vi "Axsun OCT Control Example - revise.vi"() -> ()   [LabVIEW 2018]
uses:
  C:/Users/BoasLab/Downloads/AxsunOCTControlExampleSourceCode_LabVIEW/AxsunOCTControl.dll
  AxsunOCTControl.dll
panel:
  out "BytesSent":i32
  out "TimeTaken":i32
  out "PacketsSent":i32
  out "DataBytes":i32
  out "StatusArray":u32[](array[numeric])
  out "StatusWordsReturned":u32
  out "SerialNum":string
  out "SourceCurrentOn 2":u32
  out "LaserOnTimeSeconds":u32
  in  "GetSerialNum":bool
  in  "CloseConnection":bool
  in  "GetLastCommandInfo":bool
  in  "RebootSystem":bool
  in  "GetSystemStatus":bool
  in  "SourceCurrentOFF":bool
  in  "Initialize":bool
  in  "SourceCurrentOn":bool
  out "wavelength":dbl
  in  "GetWaveLengthAtSweepTrigger":bool
  in  "GetLaserOnTime":bool
  out "Devices":string[](array[string])
  in  "Laser Off":bool
  in  "Laser On":bool
  in  "stop":bool
  out "Error":errorcluster
  out "Version":string
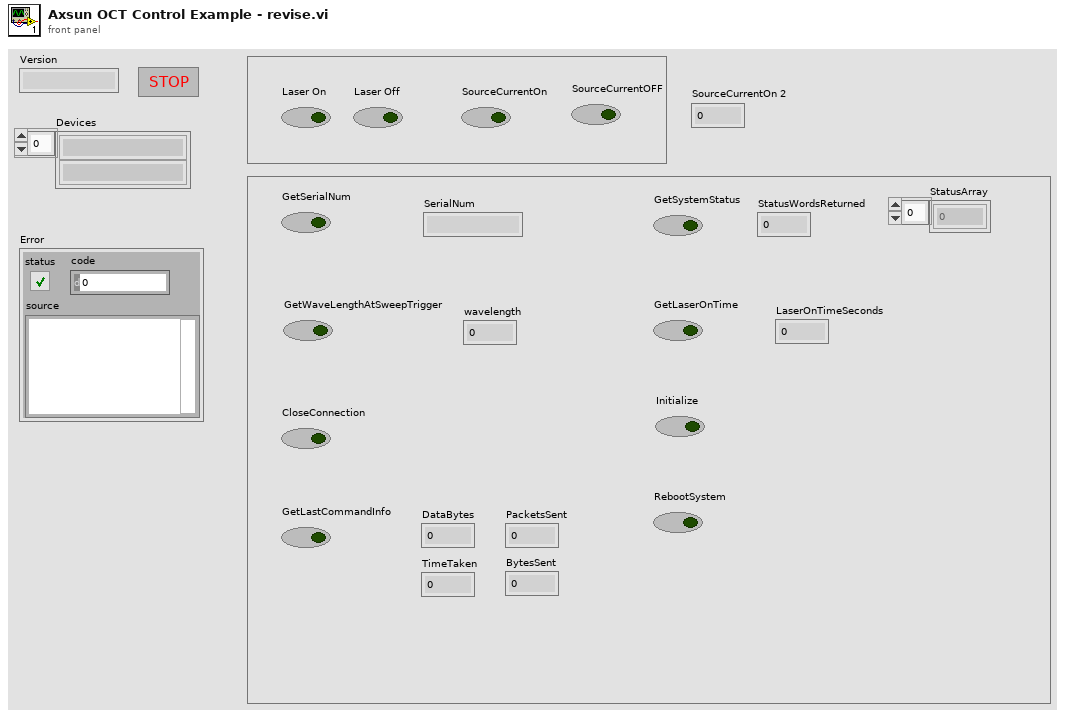
[diagram p1: front panel]
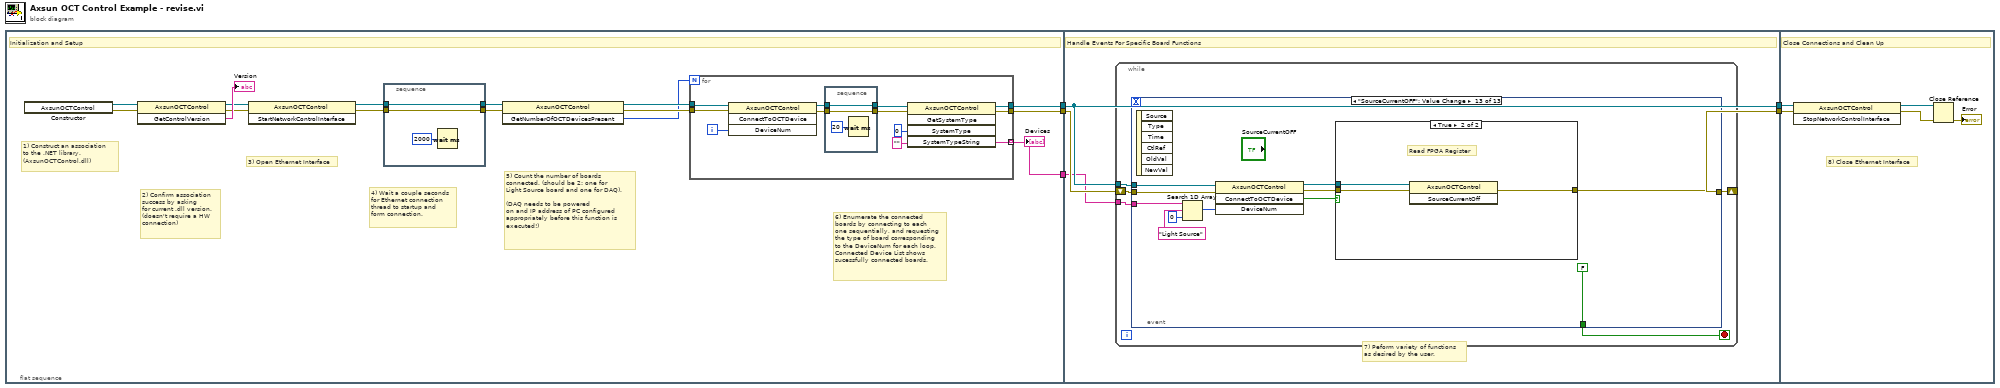
[diagram p0: block diagram]
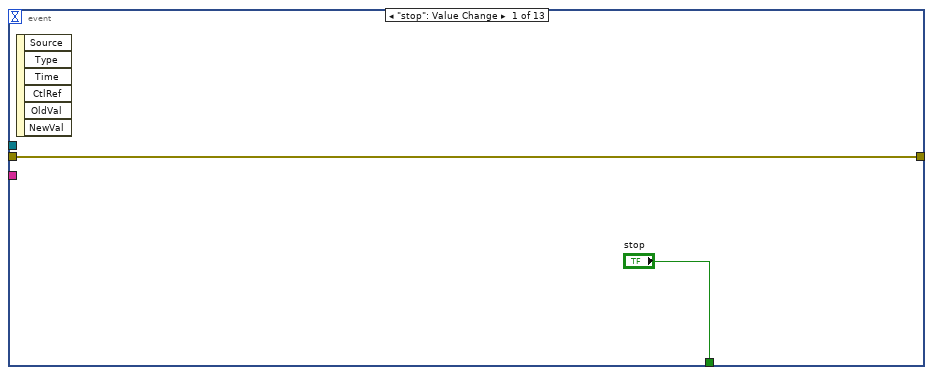
[diagram p2: hidden frame]
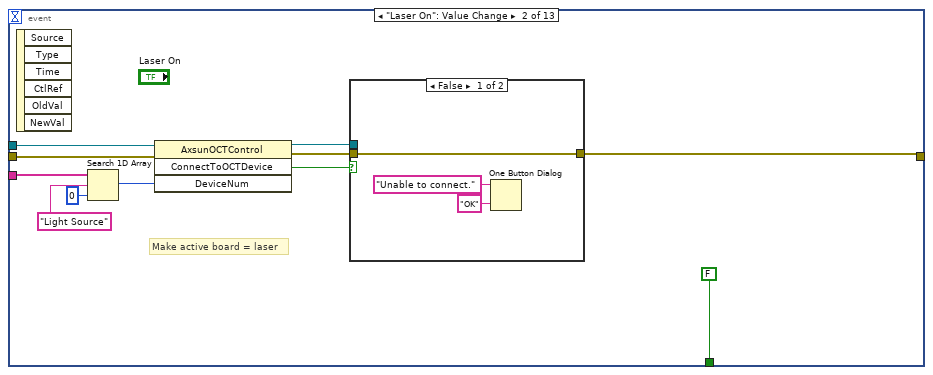
[diagram p3: hidden frame]
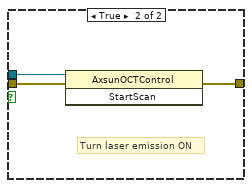
[diagram p4: hidden frame]
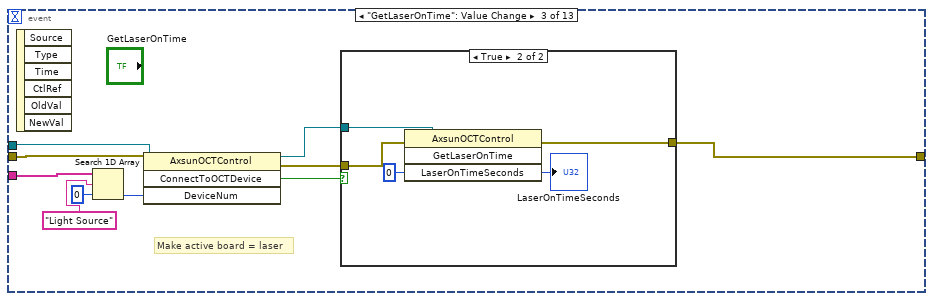
[diagram p5: hidden frame]
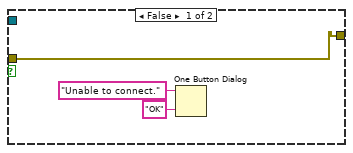
[diagram p6: hidden frame]
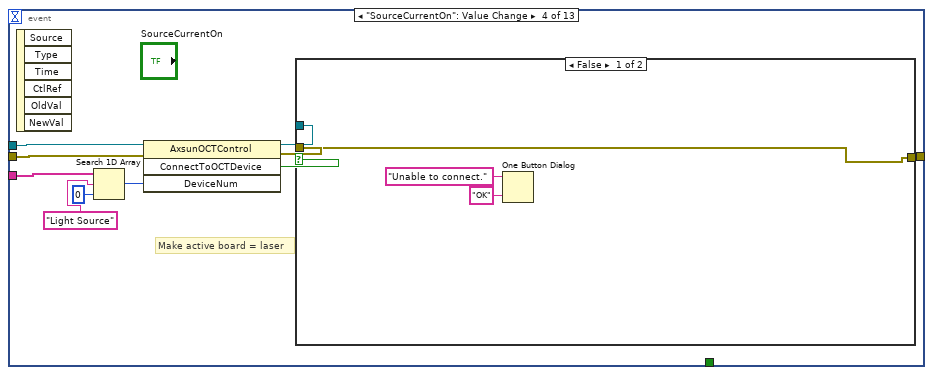
[diagram p7: hidden frame]
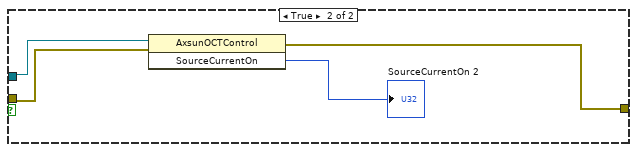
[diagram p8: hidden frame]
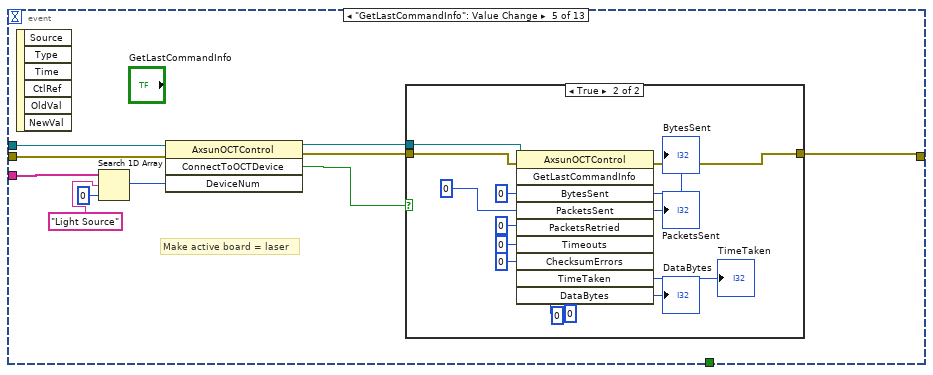
[diagram p9: hidden frame]
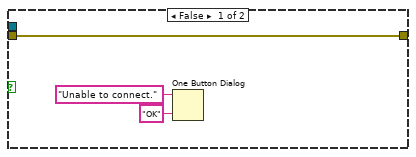
[diagram p10: hidden frame]
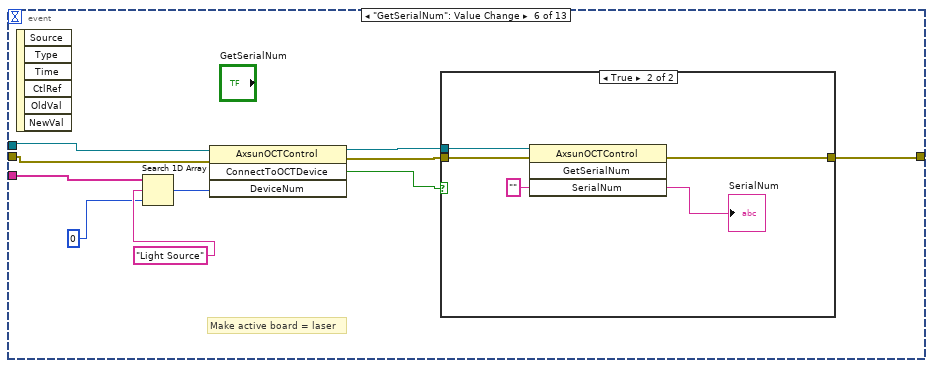
[diagram p11: hidden frame]
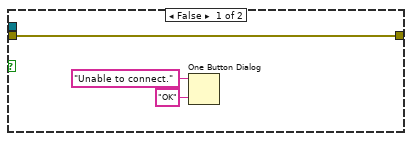
[diagram p12: hidden frame]
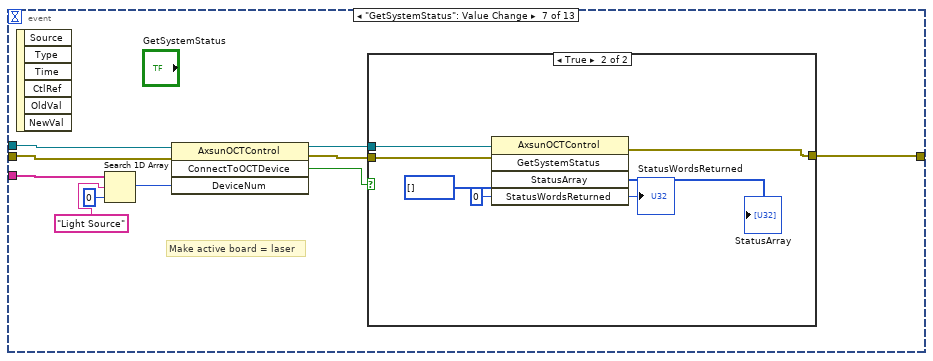
[diagram p13: hidden frame]
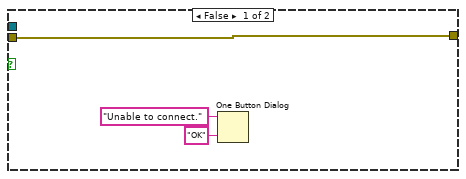
[diagram p14: hidden frame]
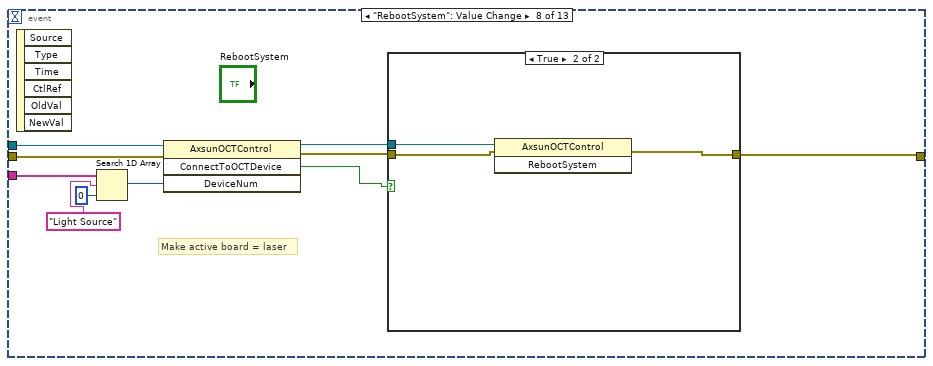
[diagram p15: hidden frame]
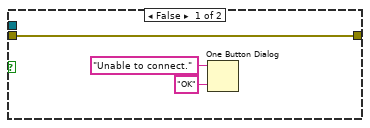
[diagram p16: hidden frame]
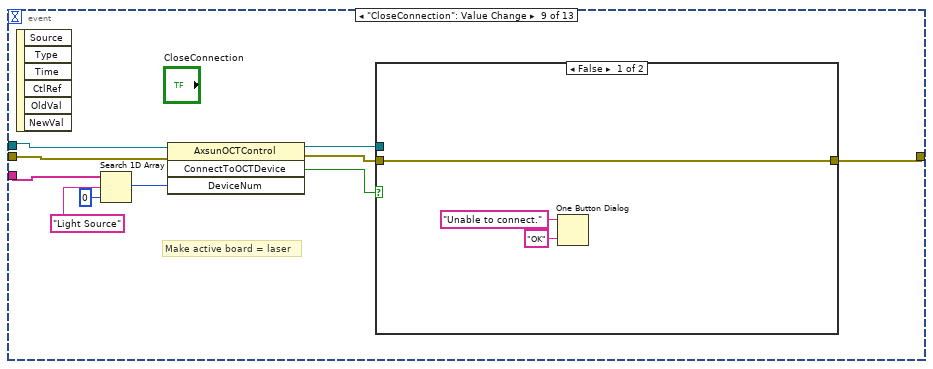
[diagram p17: hidden frame]
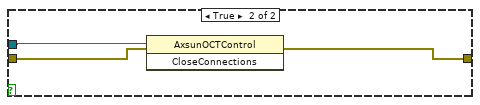
[diagram p18: hidden frame]
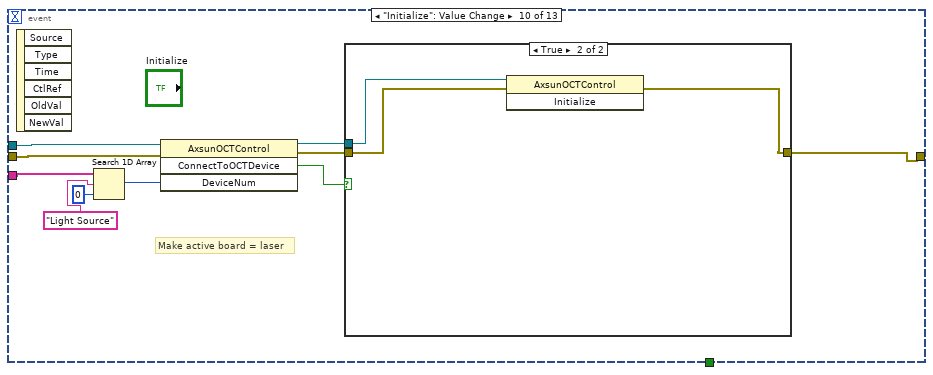
[diagram p19: hidden frame]
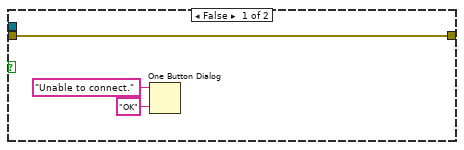
[diagram p20: hidden frame]
diagram:
  n1 = flat-sequence {
    tunnel: [w11] -> w5
    tunnel: [w10] -> w4
    tunnel: [w9] -> w2
    tunnel: w5 -> [w42]
    tunnel: w4 -> [w41]
    tunnel: [w41] -> w3
    tunnel: w2 -> [w40]
    tunnel: [w39] -> w1
    tunnel: w3 -> [w270]
    tunnel: w1 -> [w266]
    frame #0 {
      # "6) Enumerate the connected\nboards by connecting to each\none sequentially, and requesting\nthe type of board corresponding\nto the DeviceNum for each loop.\nConnected Device List shows\nsucessfully connected boards."
      # "5) Count the number of boards\nconnected. (should be 2: one for\nLight Source board and one for DAQ).\n\n(DAQ needs to be powered\non and IP address of PC configured \nappropriately before this function is\nexecuted!)"
      # "4) Wait a couple seconds\nfor Ethernet connection\nthread to startup and\nform connection."
      # "3) Open Ethernet Interface"
      # "2) Confirm association\nsuccess by asking\nfor current .dll version.\n(doesn't require a HW\nconnection)"
      # "1) Construct an association \nto the .NET library.\n(AxsunOCTControl.dll)"
      # "Initialization and Setup"
      n2 = constructor class="AxsunOCTControl"() -> (reference out=w7:refnum<k24>, error out=w6:errorcluster)  [unwired: 3 in, 1 out]
      n3 = invoke class="AxsunOCTControl" method="GetControlVersion"(reference=w7, error in=w6) -> (reference out=w19:refnum<k24>, error out=w18:errorcluster, "GetControlVersion"=→"Version":string)  [unwired: 1 in]
      n4 = invoke class="AxsunOCTControl" method="StartNetworkControlInterface"(reference=w19, error in=w18) -> (reference out=w8:refnum<k24>, error out=w17:errorcluster)  [unwired: 1 in, 1 out]
      n5 = stacked-sequence {
        tunnel: [w38] -> w16
        tunnel: w8 -> [w38]
        tunnel: [w37] -> w15
        tunnel: w17 -> [w37]
        frame #0 {
          n6 = Wait (ms)(milliseconds to wait=u32 2000) -> ()  [unwired: 1 out]
        }
      }
      n7 = invoke class="AxsunOCTControl" method="GetNumberOfOCTDevicesPresent"(reference=w16, error in=w15) -> (reference out=w14:refnum<k24>, error out=w13:errorcluster, "GetNumberOfOCTDevicesPresent"=w12:i32)  [unwired: 1 in]
      n8 = for {
        N: w12 -> [_]
        tunnel: w14 -> [w32]
        tunnel: w13 -> [w31]
        tunnel: [w27] -> w10
        tunnel: [w26] -> w11
        tunnel: [w23] -> w9 mode=indexing
        i -> [w30]
        n9 = invoke class="AxsunOCTControl" method="ConnectToOCTDevice"(reference=w32, error in=w31, "DeviceNum"=w30) -> (reference out=w25:refnum<k24>, error out=w24:errorcluster)  [unwired: 1 in, 2 out]
        n10 = stacked-sequence {
          tunnel: w25 -> [w35]
          tunnel: [w35] -> w22
          tunnel: w24 -> [w34]
          tunnel: [w34] -> w21
          frame #0 {
            n11 = Wait (ms)(milliseconds to wait=u32 20) -> ()  [unwired: 1 out]
          }
        }
        n12 = invoke class="AxsunOCTControl" method="GetSystemType"(reference=w22, error in=w21, "SystemType"=u32 0, "SystemTypeString"="") -> (reference out=w27:refnum<k24>, error out=w26:errorcluster, "SystemTypeString"=w23:string)  [unwired: 1 in, 2 out]
      }
      "Devices" <- w9
    }
    frame #1 {
      # "7) Peform variety of functions\nas desired by the user."
      # "Handle Events For Specific Board Functions"
      n13 = while {
        tunnel: w41 -> [w47]
        tunnel: w40 -> [w44]
        shift-right: [w43] -> w39
        shift-left: w42 -> [w46]
        stop <- w45 stop-if-true
        n14 = event shown="[12] \"SourceCurrentOFF\": Value Change" {
          selector: _ -> [_ _ _ _ _ _ _ _ _ _ _ _ _]
          dyn-events: _ -> [_ _ _ _ _ _ _ _ _ _ _ _ _]
          timeout: _ -> [_ _ _ _ _ _ _ _ _ _ _ _ _]
          tunnel: w47 -> [_ w57 w72 w90 w108 w133 w152 w172 w188 w202 w218 w239 w256]
          tunnel: w46 -> [w48 w56 w73 w91 w107 w134 w151 w171 w187 w203 w219 w238 w255]
          tunnel: ["stop" FALSE ("stop") _ _ _ _ _ _ _ _ _ FALSE ("stop") FALSE ("stop")] -> w45
          tunnel: w44 -> [_ w59 w71 w89 w106 w135 w150 w170 w186 w204 w220 w241 w258]
          tunnel: [w48 w52 w67 w85 w103 w128 w146 w168 w182 w198 w214 w234 w251] -> w43
          event "stop": Value Change {
            n15 = event-data() -> ()  [unwired: 1 in, 6 out]
          }
          event "Laser On": Value Change {
            # "Make active board = laser"
            n16 = event-data() -> ()  [unwired: 1 in, 6 out]
            n17 = Search 1D Array(1D array=w59, element="Light Source", start index (0)=0) -> (index of element=w55:i32)
            n18 = invoke class="AxsunOCTControl" method="ConnectToOCTDevice"(reference=w57, error in=w56, "DeviceNum"=w55) -> (reference out=w54:refnum<k24>, error out=w53:errorcluster, "ConnectToOCTDevice"=w51:bool)  [unwired: 1 in, 1 out]
            n19 = case shown="False" w51 {
              tunnel: w54 -> [_ w66]
              tunnel: w53 -> [w63 w65]
              tunnel: [w63 w64] -> w52
              frame False {
                n20 = One Button Dialog(message="Unable to connect.", button name ("OK")="OK") -> ()  [unwired: 1 out]
              }
              frame True {
                # "Turn laser emission ON"
                n21 = invoke class="AxsunOCTControl" method="StartScan"(reference=w66, error in=w65) -> (error out=w64:errorcluster)  [unwired: 1 in, 2 out]
              }
            }
          }
          event "GetLaserOnTime": Value Change {
            # "Make active board = laser"
            n22 = event-data() -> ()  [unwired: 1 in, 6 out]
            n23 = Search 1D Array(1D array=w71, element="Light Source", start index (0)=0) -> (index of element=w76:i32)
            n24 = invoke class="AxsunOCTControl" method="ConnectToOCTDevice"(reference=w72, error in=w73, "DeviceNum"=w76) -> (reference out=w69:refnum<k24>, error out=w70:errorcluster, "ConnectToOCTDevice"=w68:bool)  [unwired: 1 in, 1 out]
            n25 = case shown="True" w68 {
              tunnel: w70 -> [w79 w83]
              tunnel: w69 -> [_ w84]
              tunnel: [w79 w82] -> w67
              frame False {
                n26 = One Button Dialog(message="Unable to connect.", button name ("OK")="OK") -> ()  [unwired: 1 out]
              }
              frame True {
                n27 = invoke class="AxsunOCTControl" method="GetLaserOnTime"(reference=w84, error in=w83, "LaserOnTimeSeconds"=u32 0) -> (error out=w82:errorcluster, "LaserOnTimeSeconds"=→"LaserOnTimeSeconds":u32)  [unwired: 1 in, 2 out]
              }
            }
          }
          event "SourceCurrentOn": Value Change {
            # "Make active board = laser"
            n28 = event-data() -> ()  [unwired: 1 in, 6 out]
            n29 = Search 1D Array(1D array=w89, element="Light Source", start index (0)=0) -> (index of element=w94:i32)
            n30 = invoke class="AxsunOCTControl" method="ConnectToOCTDevice"(reference=w90, error in=w91, "DeviceNum"=w94) -> (reference out=w86:refnum<k24>, error out=w87:errorcluster, "ConnectToOCTDevice"=w88:bool)  [unwired: 1 in, 1 out]
            n31 = case shown="False" w88 {
              tunnel: w87 -> [w95 w100]
              tunnel: w86 -> [_ w101]
              tunnel: [w95 w98] -> w85
              frame False {
                n32 = One Button Dialog(message="Unable to connect.", button name ("OK")="OK") -> ()  [unwired: 1 out]
              }
              frame True {
                n33 = invoke class="AxsunOCTControl" method="SourceCurrentOn"(reference=w101, error in=w100) -> (error out=w98:errorcluster, "SourceCurrentOn"=→"SourceCurrentOn 2":u32)  [unwired: 1 in, 1 out]
              }
            }
          }
          event "GetLastCommandInfo": Value Change {
            # "Make active board = laser"
            n34 = event-data() -> ()  [unwired: 1 in, 6 out]
            n35 = Search 1D Array(1D array=w106, element="Light Source", start index (0)=0) -> (index of element=w111:i32)
            n36 = invoke class="AxsunOCTControl" method="ConnectToOCTDevice"(reference=w108, error in=w107, "DeviceNum"=w111) -> (reference out=w102:refnum<k24>, error out=w104:errorcluster, "ConnectToOCTDevice"=w105:bool)  [unwired: 1 in, 1 out]
            n37 = case shown="True" w105 {
              tunnel: w104 -> [w114 w126]
              tunnel: [w114 w125] -> w103
              tunnel: w102 -> [_ w127]
              frame False {
                n38 = One Button Dialog(message="Unable to connect.", button name ("OK")="OK") -> ()  [unwired: 1 out]
              }
              frame True {
                (unwired) 0 ("TimeTaken")
                w121 = 0 ("DataBytes")
                n39 = invoke class="AxsunOCTControl" method="GetLastCommandInfo"(reference=w127, error in=w126, "BytesSent"=0, "PacketsSent"=0, "PacketsRetried"=0, "Timeouts"=0, "ChecksumErrors"=0, "TimeTaken"=w121, "DataBytes"=w121) -> (error out=w125:errorcluster, "BytesSent"=→"BytesSent":i32, "PacketsSent"=→"PacketsSent":i32, "TimeTaken"=→"TimeTaken":i32, "DataBytes"=→"DataBytes":i32)  [unwired: 1 in, 5 out]
              }
            }
          }
          event "GetSerialNum": Value Change {
            # "Make active board = laser"
            n40 = event-data() -> ()  [unwired: 1 in, 6 out]
            n41 = Search 1D Array(1D array=w135, element="Light Source", start index (0)=0) -> (index of element=w132:i32)
            n42 = invoke class="AxsunOCTControl" method="ConnectToOCTDevice"(reference=w133, error in=w134, "DeviceNum"=w132) -> (reference out=w131:refnum<k24>, error out=w130:errorcluster, "ConnectToOCTDevice"=w129:bool)  [unwired: 1 in, 1 out]
            n43 = case shown="True" w129 {
              tunnel: w131 -> [_ w145]
              tunnel: w130 -> [w140 w144]
              tunnel: [w140 w143] -> w128
              frame False {
                n44 = One Button Dialog(message="Unable to connect.", button name ("OK")="OK") -> ()  [unwired: 1 out]
              }
              frame True {
                n45 = invoke class="AxsunOCTControl" method="GetSerialNum"(reference=w145, error in=w144, "SerialNum"="") -> (error out=w143:errorcluster, "SerialNum"=→"SerialNum":string)  [unwired: 1 in, 2 out]
              }
            }
          }
          event "GetSystemStatus": Value Change {
            # "Make active board = laser"
            n46 = event-data() -> ()  [unwired: 1 in, 6 out]
            n47 = Search 1D Array(1D array=w150, element="Light Source", start index (0)=0) -> (index of element=w155:i32)
            n48 = invoke class="AxsunOCTControl" method="ConnectToOCTDevice"(reference=w152, error in=w151, "DeviceNum"=w155) -> (reference out=w147:refnum<k24>, error out=w148:errorcluster, "ConnectToOCTDevice"=w149:bool)  [unwired: 1 in, 1 out]
            n49 = case shown="True" w149 {
              tunnel: w148 -> [w158 w164]
              tunnel: w147 -> [_ w165]
              tunnel: [w158 w159] -> w146
              frame False {
                n50 = One Button Dialog(message="Unable to connect.", button name ("OK")="OK") -> ()  [unwired: 1 out]
              }
              frame True {
                n51 = invoke class="AxsunOCTControl" method="GetSystemStatus"(reference=w165, error in=w164, "StatusArray"=u32[] [], "StatusWordsReturned"=u32 0) -> (error out=w159:errorcluster, "StatusArray"=→"StatusArray":u32[], "StatusWordsReturned"=→"StatusWordsReturned":u32)  [unwired: 1 in, 2 out]
              }
            }
          }
          event "RebootSystem": Value Change {
            # "Make active board = laser"
            n52 = event-data() -> ()  [unwired: 1 in, 6 out]
            n53 = Search 1D Array(1D array=w170, element="Light Source", start index (0)=0) -> (index of element=w175:i32)
            n54 = invoke class="AxsunOCTControl" method="ConnectToOCTDevice"(reference=w172, error in=w171, "DeviceNum"=w175) -> (reference out=w167:refnum<k24>, error out=w166:errorcluster, "ConnectToOCTDevice"=w169:bool)  [unwired: 1 in, 1 out]
            n55 = case shown="True" w169 {
              tunnel: w166 -> [w178 w180]
              tunnel: [w178 w179] -> w168
              tunnel: w167 -> [_ w181]
              frame False {
                n56 = One Button Dialog(message="Unable to connect.", button name ("OK")="OK") -> ()  [unwired: 1 out]
              }
              frame True {
                n57 = invoke class="AxsunOCTControl" method="RebootSystem"(reference=w181, error in=w180) -> (error out=w179:errorcluster)  [unwired: 1 in, 2 out]
              }
            }
          }
          event "CloseConnection": Value Change {
            # "Make active board = laser"
            n58 = event-data() -> ()  [unwired: 1 in, 6 out]
            n59 = Search 1D Array(1D array=w186, element="Light Source", start index (0)=0) -> (index of element=w189:i32)
            n60 = invoke class="AxsunOCTControl" method="ConnectToOCTDevice"(reference=w188, error in=w187, "DeviceNum"=w189) -> (reference out=w185:refnum<k24>, error out=w184:errorcluster, "ConnectToOCTDevice"=w183:bool)  [unwired: 1 in, 1 out]
            n61 = case shown="False" w183 {
              tunnel: w185 -> [_ w197]
              tunnel: w184 -> [w194 w196]
              tunnel: [w194 w195] -> w182
              frame False {
                n62 = One Button Dialog(message="Unable to connect.", button name ("OK")="OK") -> ()  [unwired: 1 out]
              }
              frame True {
                n63 = invoke class="AxsunOCTControl" method="CloseConnections"(reference=w197, error in=w196) -> (error out=w195:errorcluster)  [unwired: 1 in, 2 out]
              }
            }
          }
          event "Initialize": Value Change {
            # "Make active board = laser"
            n64 = event-data() -> ()  [unwired: 1 in, 6 out]
            n65 = Search 1D Array(1D array=w204, element="Light Source", start index (0)=0) -> (index of element=w207:i32)
            n66 = invoke class="AxsunOCTControl" method="ConnectToOCTDevice"(reference=w202, error in=w203, "DeviceNum"=w207) -> (reference out=w199:refnum<k24>, error out=w200:errorcluster, "ConnectToOCTDevice"=w201:bool)  [unwired: 1 in, 1 out]
            n67 = case shown="True" w201 {
              tunnel: w200 -> [w210 w212]
              tunnel: w199 -> [_ w213]
              tunnel: [w210 w211] -> w198
              frame False {
                n68 = One Button Dialog(message="Unable to connect.", button name ("OK")="OK") -> ()  [unwired: 1 out]
              }
              frame True {
                n69 = invoke class="AxsunOCTControl" method="Initialize"(reference=w213, error in=w212) -> (error out=w211:errorcluster)  [unwired: 1 in, 2 out]
              }
            }
          }
          event "GetWaveLengthAtSweepTrigger": Value Change {
            # "Make active board = laser"
            n70 = event-data() -> ()  [unwired: 1 in, 6 out]
            n71 = Search 1D Array(1D array=w220, element="Light Source", start index (0)=0) -> (index of element=w223:i32)
            n72 = invoke class="AxsunOCTControl" method="ConnectToOCTDevice"(reference=w218, error in=w219, "DeviceNum"=w223) -> (reference out=w216:refnum<k24>, error out=w215:errorcluster, "ConnectToOCTDevice"=w217:bool)  [unwired: 1 in, 1 out]
            n73 = case shown="True" w217 {
              tunnel: w216 -> [_ w231]
              tunnel: w215 -> [w226 w230]
              tunnel: [w226 w229] -> w214
              frame False {
                n74 = One Button Dialog(message="Unable to connect.", button name ("OK")="OK") -> ()  [unwired: 1 out]
              }
              frame True {
                n75 = invoke class="AxsunOCTControl" method="GetWavelengthAtSweepTrigger"(reference=w231, error in=w230, "Wavelength"=0.0) -> (error out=w229:errorcluster, "Wavelength"=→"wavelength":dbl)  [unwired: 1 in, 2 out]
              }
            }
          }
          event "Laser Off": Value Change {
            # "Make active board = laser"
            n76 = event-data() -> ()  [unwired: 1 in, 6 out]
            n77 = Search 1D Array(1D array=w241, element="Light Source", start index (0)=0) -> (index of element=w237:i32)
            n78 = invoke class="AxsunOCTControl" method="ConnectToOCTDevice"(reference=w239, error in=w238, "DeviceNum"=w237) -> (reference out=w236:refnum<k24>, error out=w235:errorcluster, "ConnectToOCTDevice"=w233:bool)  [unwired: 1 in, 1 out]
            n79 = case shown="True" w233 {
              tunnel: w236 -> [_ w248]
              tunnel: w235 -> [w245 w247]
              tunnel: [w245 w246] -> w234
              frame False {
                n80 = One Button Dialog(message="Unable to connect.", button name ("OK")="OK") -> ()  [unwired: 1 out]
              }
              frame True {
                # "Turn laser emission OFF"
                n81 = invoke class="AxsunOCTControl" method="StopScan"(reference=w248, error in=w247) -> (error out=w246:errorcluster)  [unwired: 1 in, 2 out]
              }
            }
          }
          event "SourceCurrentOFF": Value Change {
            n82 = event-data() -> ()  [unwired: 1 in, 6 out]
            n83 = Search 1D Array(1D array=w258, element="Light Source", start index (0)=0) -> (index of element=w254:i32)
            n84 = invoke class="AxsunOCTControl" method="ConnectToOCTDevice"(reference=w256, error in=w255, "DeviceNum"=w254) -> (reference out=w253:refnum<k24>, error out=w252:errorcluster, "ConnectToOCTDevice"=w250:bool)  [unwired: 1 in, 1 out]
            n85 = case shown="True" w250 {
              tunnel: w253 -> [_ w265]
              tunnel: w252 -> [w262 w264]
              tunnel: [w262 w263] -> w251
              frame False {
                n86 = One Button Dialog(message="Unable to connect.", button name ("OK")="OK") -> ()  [unwired: 1 out]
              }
              frame True {
                # "Read FPGA Register"
                n87 = invoke class="AxsunOCTControl" method="SourceCurrentOff"(reference=w265, error in=w264) -> (error out=w263:errorcluster)  [unwired: 1 in, 2 out]
              }
            }
          }
        }
      }
    }
    frame #2 {
      # "8) Close Ethernet Interface"
      # "Close Connections and Clean Up"
      n88 = invoke class="AxsunOCTControl" method="StopNetworkControlInterface"(reference=w270, error in=w266) -> (reference out=w269:refnum<k24>, error out=w268:errorcluster)  [unwired: 1 in, 1 out]
      n89 = Close Reference(reference=w269, error in (no error)=w268) -> (error out=→"Error":errorcluster)
    }
  }
